vi "GOOPUtil_IsInstanceOf.vi"(0 "GOOP Object":refnum<class>, 1 "Is Instance of Object":refnum<class>, 5 "error in (no error)":errorcluster) -> (14 "IsInstanceOf":bool, 19 "error out":errorcluster)   [LabVIEW 2020, in "GOOPUtility.lvlib"]
doc: "Compares if the GOOP object is an instance (or subclass) of the specified \"Is Instance of Object\".\n\nThis is a collection of generic GOOP utility VIs. Please notice that it is important that the frontpanel of the Create, Destroy and GetObjectStatus is not removed when building an application."
uses:
  GOOPUtility.lvlib
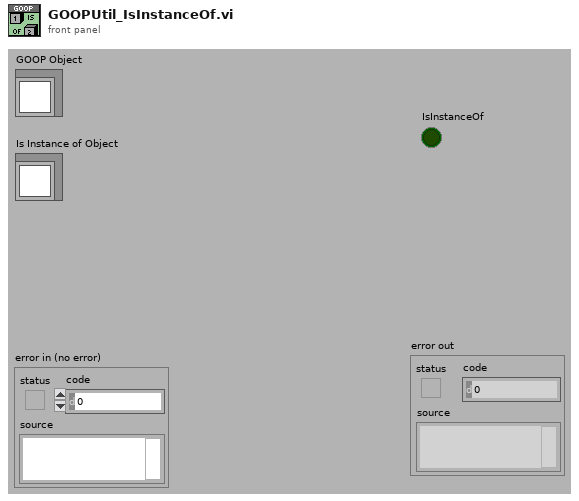
[diagram p1: front panel]
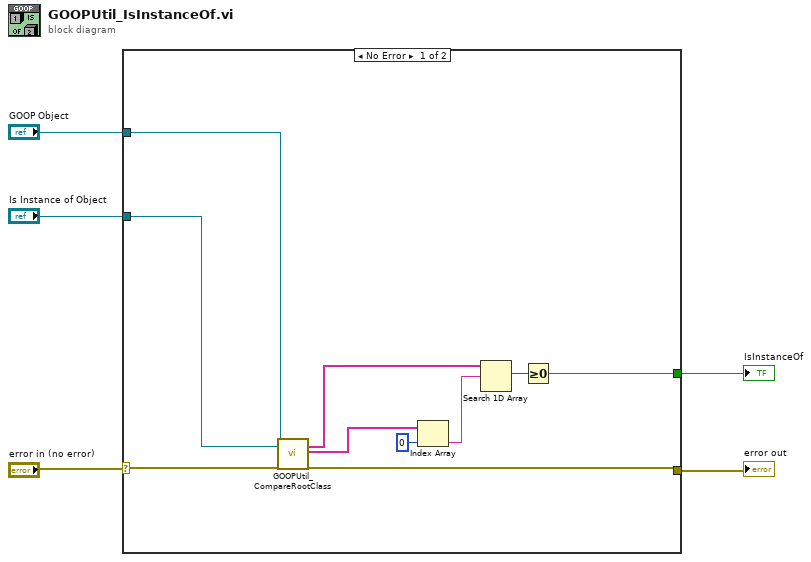
[diagram p0: block diagram]
diagram:
  n1 = case shown="No Error" "error in (no error)" {
    selector: "error in (no error)" -> [w15 w16]
    tunnel: "GOOP Object" -> [w14 _]
    tunnel: "Is Instance of Object" -> [w13 _]
    tunnel: [w9 w16] -> w2
    tunnel: [w7 _] -> w1
    frame No Error {
      n2 = call "GOOPUtil_CompareRootClass.vi"("GOOP Object 1"=w14, "GOOP Object 2"=w13, "error in (no error)"=w15) -> ("GOOPObject1Ancestors"=w10:string[], "GOOPObject2Ancestors"=w6:string[], "error out"=w9:errorcluster)  [unwired: 13 in, 1 out]
      n3 = Index Array(array=w6, index=0) -> (element=w11:string)
      n4 = Search 1D Array(1D array=w10, element=w11) -> (index of element=w8:i32)  [unwired: 1 in]
      n5 = Greater Or Equal To 0?(x=w8) -> (x >= 0?=w7:bool)
    }
    frame Error {
    }
  }
  "error out" <- w2
  "IsInstanceOf" <- w1
